vi "Time Stamp To Integer.vi"(7 "time format string (%c)":string="%Y%m%d%H%M%S", 10 "Time Stamp In":timestamp format="%<%.3X %x>T") -> (2 "Integer Out":i64)   [LabVIEW 2024]
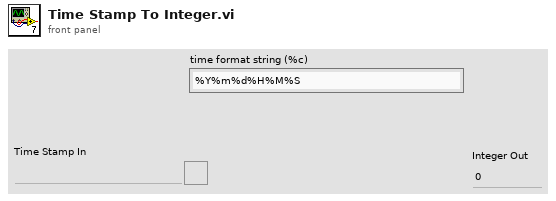
[diagram p1: front panel]
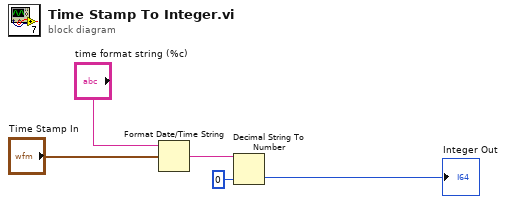
[diagram p0: block diagram]
diagram:
  n1 = Format Date/Time String(time format string (%c)="time format string (%c)", seconds (now)="Time Stamp In") -> (date/time string=w3:string)  [unwired: 1 in]
  n2 = Decimal String To Number(string=w3, default (0L)=i64 0 ("default (0 I32)")) -> (number=→"Integer Out":i64)  [unwired: 1 in, 1 out]
